vi "MotorMath.vi"(8 "Motor velocity":dbl) -> (0 "output cluster":cluster{i32, "upper limit":dbl})   [LabVIEW 2012]
panel:
  in  "10% speed (RPM)":dbl=-5000.0
  in  "90% speed (RPM)":dbl=5000.0
  # "Maximum and minimum speeds defined by Maxon controller"
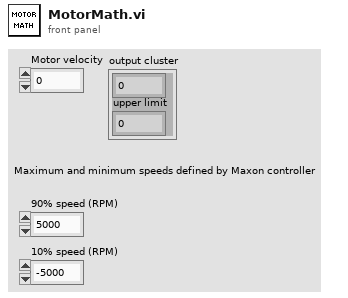
[diagram p1: front panel]
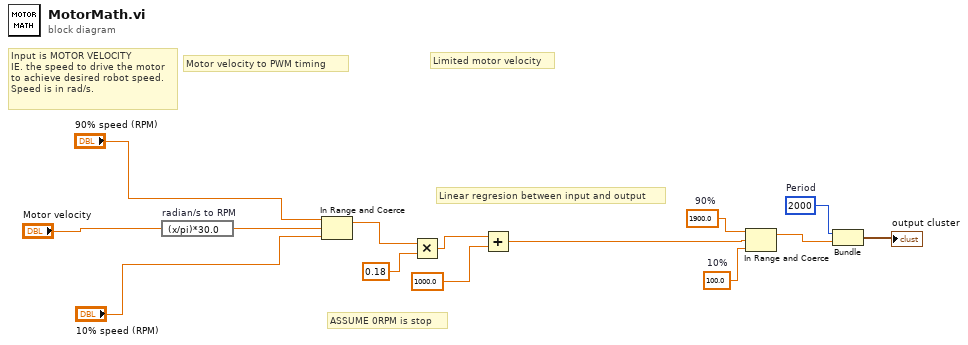
[diagram p0: block diagram]
diagram:
  w6 = 100.0  # 10%
  w7 = 1900.0  # 90%
  w14 = 2000  # Period
  # "Linear regresion between input and output"
  # "ASSUME 0RPM is stop"
  # "Limited motor velocity"
  # "Input is MOTOR VELOCITY\nIE. the speed to drive the motor\nto achieve desired robot speed.\nSpeed is in rad/s."
  # "Motor velocity to PWM timing"
  n1 = expression code="(x/pi)*30.0" "radian/s to RPM"("Motor velocity") -> (w1:dbl)
  n2 = In Range and Coerce(upper limit="90% speed (RPM)", x=w1, lower limit="10% speed (RPM)") -> (coerced(x)=w12:dbl)  [unwired: 1 out]
  n3 = Multiply(x=w12, y=0.18) -> (x*y=w10:dbl)
  n4 = Add(x=w10, y=1000.0) -> (x+y=w8:dbl)
  n5 = In Range and Coerce(upper limit=w7, x=w8, lower limit=w6) -> (coerced(x)=w5:dbl)  [unwired: 1 out]
  n6 = Bundle("Period"=w14, "90%"=w5) -> (→"output cluster":cluster{"Period":i32, "90%":dbl})  [unwired: 1 in]
